vi "highScores.vi"(8 "error in (no error)":errorcluster, 9 "High Scores":map{string, i32}(c390), 11 "simonMessages in":refnum<class "simonMessages.lvclass">) -> (0 "error out":errorcluster, 3 "simonMessages out":refnum<class "simonMessages.lvclass">)   [LabVIEW 2020, in "simonMessages.lvclass"]
uses:
  simonMessages.lvclass
  simonMessages.lvclass/simonMessages.ctl
  b6e58612-9e71-409f-953b-b31247882378.vi
  <vilib>/Array/Sort 2D Array - Pop Stack.vi
  <vilib>/Array/Sort 2D Array - Push Stack.vi
  TextDisplay/TextDisplay Class.lvclass
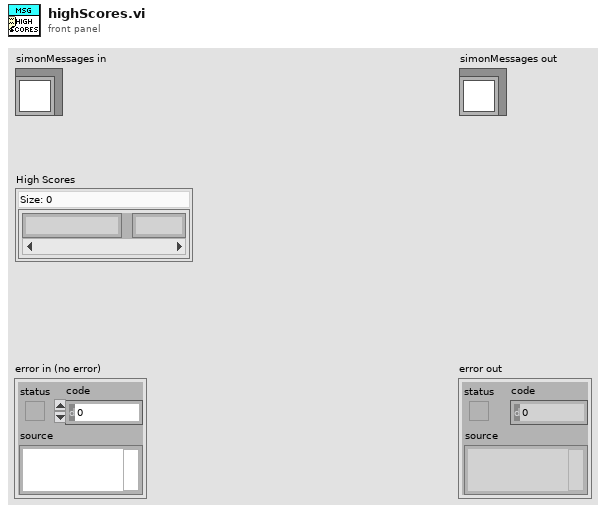
[diagram p1: front panel]
types:
  T1 = map{string, cluster{"Text":string, "Size":u8, "Justification":enum16{"Left", "Center", "Right"}, "Display Type":string}}
  T2 = cluster{"Text":string, "Size":u8, "Justification":enum16{"Left", "Center", "Right"}, "Display Type":string}
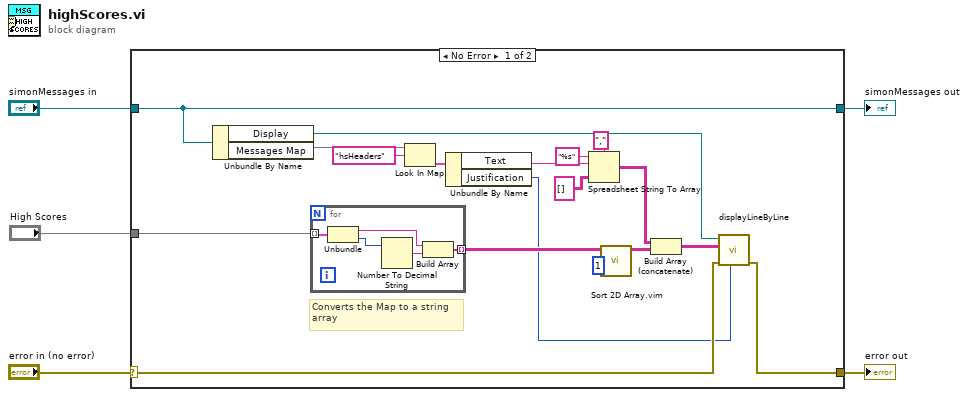
[diagram p0: block diagram]
diagram:
  n1 = case shown="No Error" "error in (no error)" {
    selector: "error in (no error)" -> [w17 w30]
    tunnel: [w18 w30] -> w4
    tunnel: [w16 w29] -> w2
    tunnel: "simonMessages in" -> [w16 w29]
    tunnel: "High Scores" -> [w19 _]
    frame No Error {
      # "Converts the Map to a string\narray"
      n2 = Unbundle By Name(w16) -> ("Display"=w15:refnum<class "TextDisplay Class.lvclass">, "Messages Map"=w14:T1)
      n3 = for {
        tunnel: w19 -> [w28] mode=indexing
        tunnel: [w24] -> w21 mode=indexing
        n4 = Unbundle(w28) -> (w25:string, w27:i32)
        n5 = Number To Decimal String(number=w27) -> (decimal integer string=w26:string)  [unwired: 1 in]
        n6 = Build Array(w25, w26) -> (w24:string[])
      }
      n7 = Look In Map(map=w14, key="hsHeaders") -> (value=w12:T2)  [unwired: 1 in, 1 out]
      n8 = Unbundle By Name(w12) -> ("Text"=w7:string, "Justification"=w6:enum16{"Left", "Center", "Right"})
      n9 = Spreadsheet String To Array(delimiter (Tab)=",", format string="%s", spreadsheet string=w7, array type (2D Dbl)=string[][] [] ("scoreLog")) -> (array=w8:string[][])
      n10 = call "Sort 2D Array.vim"("index"=1, "2D array"=w21) -> ("sorted 2D array"=w23:string[][])  [unwired: 8 in, 1 out]
      n11 = Build Array (concatenate)(w8, w23) -> (w22:string[][])
      n12 = call "displayLineByLine.vi"("Justification"=w6, "error in (no error)"=w17, "scoreLog"=w22, "TextDisplay Class in"=w15) -> ("error out"=w18:errorcluster)  [unwired: 6 in, 1 out]
    }
    frame Error {
    }
  }
  "error out" <- w4
  "simonMessages out" <- w2
